vi "Autocalc Octree resolution.vi"(1 "Triangles array":T1[](array[typedef])) -> (0 "Suggested resolution":sgl)   [LabVIEW 2014]
uses:
  Typedefs/Triangle.ctl
panel:
  # "PN 20/01/2015"
  # "Vertices"
  # "Edges"
  # "Unit normal"
  # "pre-store"
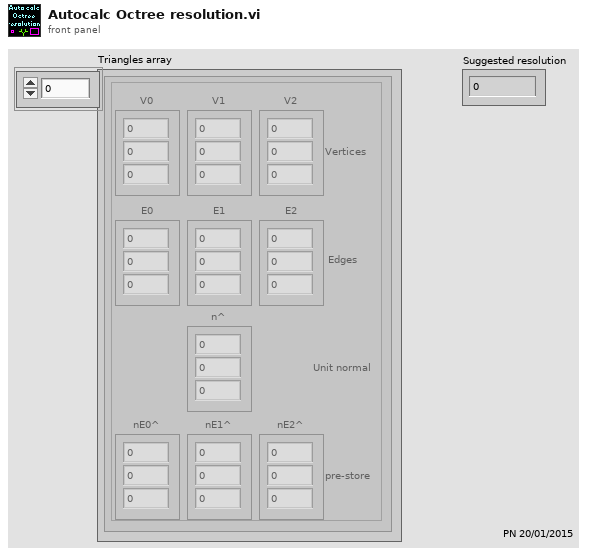
[diagram p1: front panel]
types:
  T1 = typedef "Triangle.ctl" = cluster{"V0":sgl[], "V1":sgl[], "V2":sgl[], "E0":sgl[], "E1":sgl[], "E2":sgl[], "n^":sgl[], "nE0^":sgl[], "nE1^":sgl[], "nE2^":sgl[]}
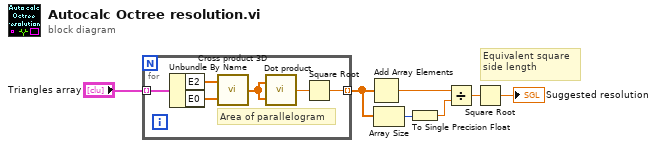
[diagram p0: block diagram]
diagram:
  # "Equivalent square side length"
  n1 = for {
    tunnel: "Triangles array" -> [w11] mode=indexing
    tunnel: [w8] -> w1 mode=indexing
    # "Area of parallelogram"
    n2 = Unbundle By Name(w11) -> ("E2"=w10:sgl[], "E0"=w9:sgl[])
    n3 = call "Cross product 3D.vi"("B"=w9, "A"=w10) -> ("A x B"=w12:sgl[])
    n4 = call "Dot product.vi"("B"=w12, "A"=w12) -> ("A . B"=w13:sgl)
    n5 = Square Root(x=w13) -> (sqrt(x)=w8:sgl)
  }
  n6 = Add Array Elements(numeric array=w1) -> (sum=w6:sgl)
  n7 = Array Size(array=w1) -> (size(s)=w5:i32)
  n8 = To Single Precision Float(number=w5) -> (single precision float=w7:sgl)
  n9 = Divide(x=w6, y=w7) -> (x/y=w2:sgl)
  n10 = Square Root(x=w2) -> (sqrt(x)=→"Suggested resolution":sgl)
